vi "Mix Columns4.vi"(11 "State In":u16[][](array[numeric])) -> (3 "数组":u16[][](array[numeric]))   [LabVIEW 2016, in "数据传输系统.lvlib"]
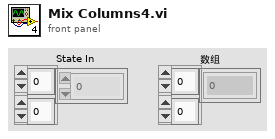
[diagram p1: front panel]
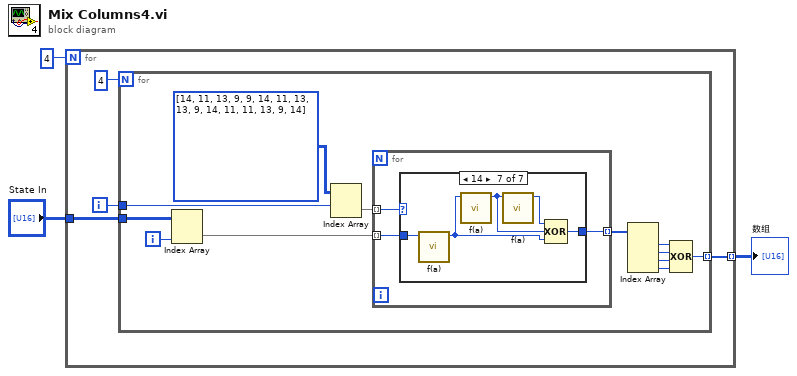
[diagram p0: block diagram]
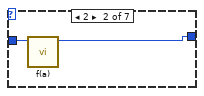
[diagram p3: hidden frame]
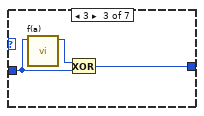
[diagram p4: hidden frame]
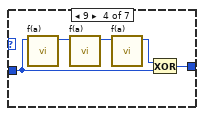
[diagram p5: hidden frame]
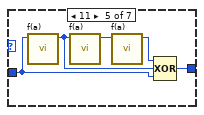
[diagram p6: hidden frame]
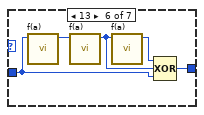
[diagram p7: hidden frame]
diagram:
  n1 = for {
    N: 4 -> [_]
    tunnel: "State In" -> [w7]
    tunnel: [w4] -> w2 mode=indexing
    i -> [w5]
    n2 = for {
      N: 4 -> [_]
      tunnel: w7 -> [w19]
      tunnel: w5 -> [w9]
      tunnel: [w11] -> w4 mode=indexing
      i -> [w10]
      n3 = Index Array(array=w19, index (col)=w10) -> (element=w18:u16[])  [unwired: 1 in]
      n4 = Index Array(array=i32[][] [[14, 11, 13, 9], [9, 14, 11, 13], [13, 9, 14, 11], [11, 13, 9, 14]] ("t[c]"), index (row)=w9) -> (element=w17:i32[])  [unwired: 1 in]
      n5 = for {
        tunnel: w18 -> [w22] mode=indexing
        tunnel: w17 -> [w21] mode=indexing
        tunnel: [w20] -> w16 mode=indexing
        n6 = case shown="14" w21 {
          tunnel: w22 -> [w23 w25 w27 w30 w35 w41 w47]
          tunnel: [w23 w24 w26 w29 w34 w40 w46] -> w20
          frame 1, Default {
          }
          frame 2 {
            n7 = call "f(a).vi"("x"=w25) -> ("数值"=w24:u16)  [unwired: 10 in]
          }
          frame 3 {
            n8 = call "f(a).vi"("x"=w27) -> ("数值"=w28:u16)  [unwired: 10 in]
            n9 = Exclusive Or(1:w27, 2:w28) -> (0:w26:u16)
          }
          frame 9 {
            n10 = call "f(a).vi"("x"=w30) -> ("数值"=w33:u16)  [unwired: 10 in]
            n11 = call "f(a).vi"("x"=w33) -> ("数值"=w32:u16)  [unwired: 10 in]
            n12 = call "f(a).vi"("x"=w32) -> ("数值"=w31:u16)  [unwired: 10 in]
            n13 = Exclusive Or(1:w30, 2:w31) -> (0:w29:u16)
          }
          frame 11 {
            n14 = call "f(a).vi"("x"=w35) -> ("数值"=w36:u16)  [unwired: 10 in]
            n15 = call "f(a).vi"("x"=w36) -> ("数值"=w38:u16)  [unwired: 10 in]
            n16 = call "f(a).vi"("x"=w38) -> ("数值"=w37:u16)  [unwired: 10 in]
            n17 = Compound Arithmetic op=XOR(w37, w36, w35) -> (w34:u16)
          }
          frame 13 {
            n18 = call "f(a).vi"("x"=w41) -> ("数值"=w42:u16)  [unwired: 10 in]
            n19 = call "f(a).vi"("x"=w42) -> ("数值"=w39:u16)  [unwired: 10 in]
            n20 = call "f(a).vi"("x"=w39) -> ("数值"=w43:u16)  [unwired: 10 in]
            n21 = Compound Arithmetic op=XOR(w43, w39, w41) -> (w40:u16)
          }
          frame 14 {
            n22 = call "f(a).vi"("x"=w47) -> ("数值"=w44:u16)  [unwired: 10 in]
            n23 = call "f(a).vi"("x"=w44) -> ("数值"=w45:u16)  [unwired: 10 in]
            n24 = call "f(a).vi"("x"=w45) -> ("数值"=w48:u16)  [unwired: 10 in]
            n25 = Compound Arithmetic op=XOR(w48, w45, w44) -> (w46:u16)
          }
        }
      }
      n26 = Index Array(array=w16) -> (element #1=w15:u16, element #2=w14:u16, element #3=w13:u16, element #4=w12:u16)  [unwired: 4 in]
      n27 = Compound Arithmetic op=XOR(w15, w14, w13, w12) -> (w11:u16)
    }
  }
  "数组" <- w2
